vi "OverlayBitmap.vi"   [LabVIEW 2024, in "OpenLvVision_Overlays.lvlib"]
doc: "Overlays an bitmap on top of an image."
uses:
  OpenLvVision_Overlays.lvlib
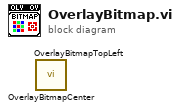
[diagram p0: block diagram]
diagram:
  n1 = call "OverlayBitmapCenter.vi"() -> ()  [unwired: 10 in, 2 out]
  n2 = call "OverlayBitmapTopLeft.vi"() -> ()  [unwired: 10 in, 2 out]
